vi "CreateParametricWaveform.vi"(1 "Description":string, 3 "error in (no error)":errorcluster, 4 "Attribute":u16(ring) items=["Not Predefined", "Predefined"], 5 "Param. Wave Name":string, 6 "VISA resource name":refnum<visa-resource-name>) -> (0 "error out":errorcluster, 2 "VISA resource name out":refnum<visa-resource-name>)   [LabVIEW 2020, in "Active Technologies AWG3000.lvlib"]
uses:
  Active Technologies AWG3000.lvlib
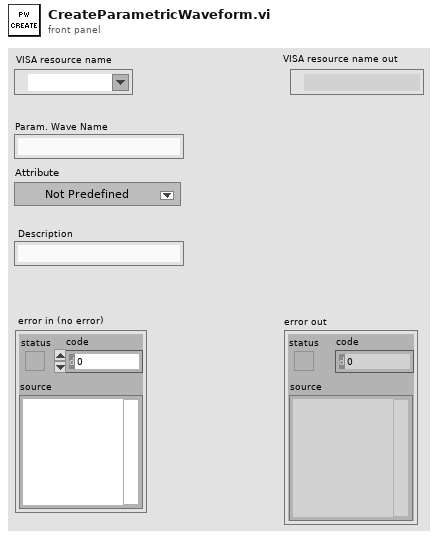
[diagram p1: front panel]
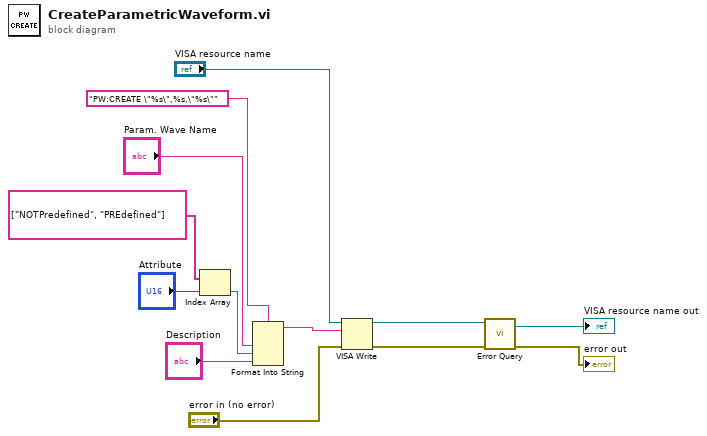
[diagram p0: block diagram]
diagram:
  n1 = Index Array(array=string[] ["NOTPredefined", "PREdefined"], index="Attribute") -> (element=w2:string)
  n2 = Format Into String(format string="PW:CREATE \"%s\",%s,\"%s\"" ("write buffer"), "Param. Wave Name", w2, "Description") -> (resulting string=w7:string)  [unwired: 2 in, 1 out]
  n3 = VISA Write(VISA resource name="VISA resource name", write buffer=w7, error in (no error)="error in (no error)") -> (VISA resource name out=w11:refnum<visa-resource-name>, error out=w10:errorcluster)  [unwired: 1 out]
  n4 = call "Error Query.vi"("error in (no error)"=w10, "VISA resource name"=w11) -> ("error out"=→"error out":errorcluster, "VISA resource name out"=→"VISA resource name out":refnum<visa-resource-name>)  [unwired: 6 in, 2 out]
